vi "MGCC_ProtCoord_main.vi"   [LabVIEW 2016]
doc: "-----------------------------------------------------------------------------------------------------------------------\nCopyright <2019> <The University of Tennessee at Knoxville and the University of Tennessee Research Foundation>\nThis software is released under BSD-3 \nhttps://opensource.org/licenses/BSD-3-Clause \nAdditional license options available at https://utrf.tennessee.edu/industry/sample-agreements/\n-----------------------------------------------------------------------------------------------------------------------"
uses:
  <vilib>/imath/engines/lvmath2/RunTimeEngine/VariableToken/NIMS_VariableToken_CondDefined.vi
  <vilib>/imathl/engines/lvmath/Functions/Error Handling/Create Error.vi
  <vilib>/imath/engines/lvmath2/RunTimeEngine/NodeEndStatement/NIMS_NodeEndStatement_Output.vi
  <vilib>/imath/engines/lvmath2/RunTimeEngine/ErrorHandling/NIMS_Finalize Error.vi
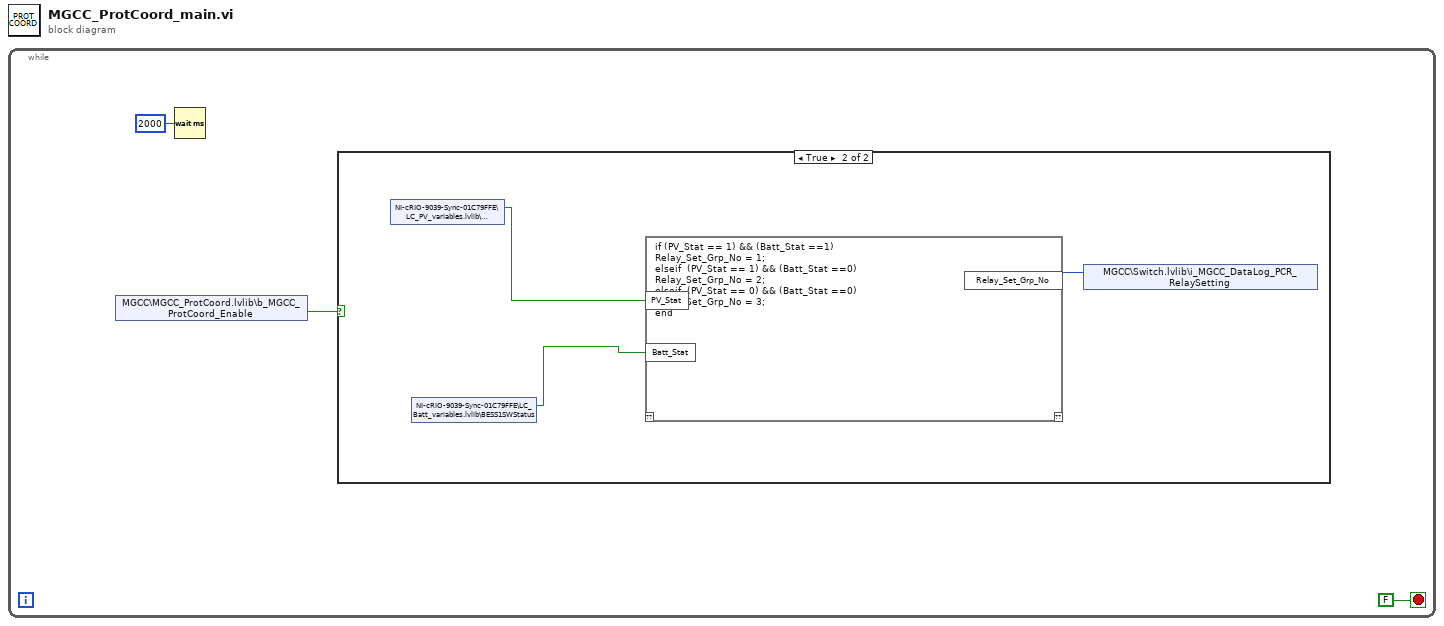
[diagram p0: block diagram]
diagram:
  n1 = while {
    stop <- FALSE stop-if-true
    n2 = shared-variable "MGCC\\MGCC_ProtCoord.lvlib\\b_MGCC_ProtCoord_Enable"() -> (w3:bool)  [unwired: 1 in, 1 out]
    n3 = Wait (ms)(milliseconds to wait=u32 2000) -> ()  [unwired: 1 out]
    n4 = case shown="True" w3 {
      frame False {
      }
      frame True {
        n5 = shared-variable "NI-cRIO-9039-Sync-01C79FFE\\LC_PV_variables.lvlib\\PV1SWStatus"() -> (w5:bool)  [unwired: 1 in, 1 out]
        n6 = shared-variable "NI-cRIO-9039-Sync-01C79FFE\\LC_Batt_variables.lvlib\\BESS1SWStatus"() -> (w4:bool)  [unwired: 1 in, 1 out]
        n7 = mathscript code="if (PV_Stat == 1) && (Batt_Stat ==1)\nRelay_Set_Grp_No = 1;\nelseif  (PV_Stat == 1) && (Batt_Stat ==0)\nRelay_Set_Grp_No = 2;\nelseif  (PV_Stat == 0) && (Batt_Stat ==0)\nRelay_Set_Grp_No = 3;\nend"("PV_Stat"=w5, "Batt_Stat"=w4) -> ("Relay_Set_Grp_No"=w6:i32)  [unwired: 1 in, 1 out]
        n8 = shared-variable "MGCC\\Switch.lvlib\\i_MGCC_DataLog_PCR_RelaySetting"(w6) -> ()  [unwired: 1 in, 1 out]
      }
    }
  }
